vi "set ignition.vi"(10 "Ignition":bool, 11 "Array":T1[](array[typedef]) {"Data" format="%.0x"}) -> (3 "Array 2":T1[](array[typedef]) {"Data" format="%.0x"})   [LabVIEW 2021, in "uCanDriver.lvlib" / "uCAN.lvclass"]
uses:
  uCAN.lvclass
  typedefs/frame.ctl
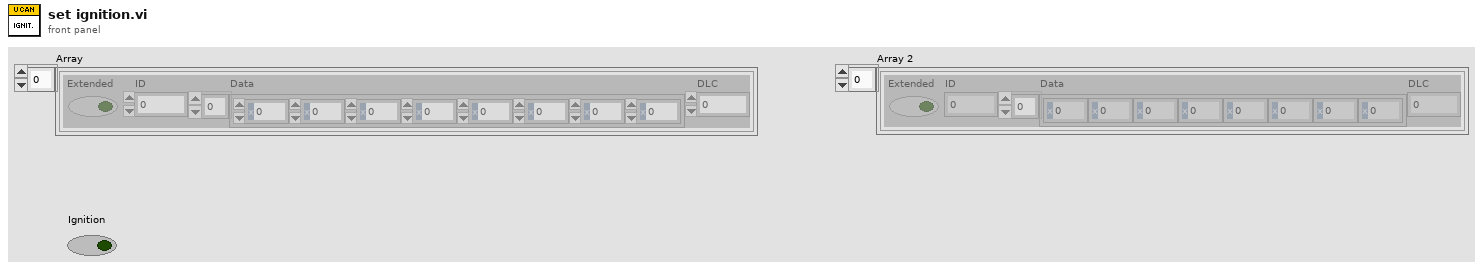
[diagram p1: front panel]
types:
  T1 = typedef "uCanDriver.lvlib/uCAN.lvclass/frame.ctl" = cluster{"Extended":bool, "ID":u32, "Data":u8[], "DLC":u8}
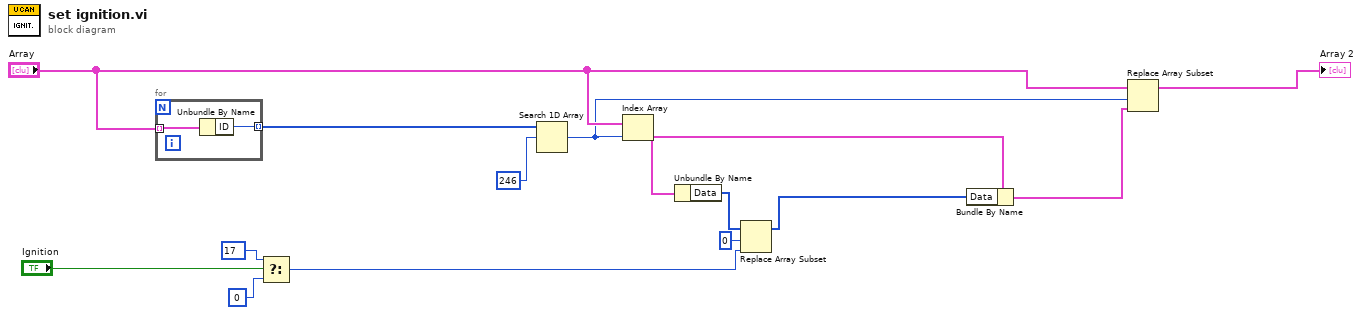
[diagram p0: block diagram]
diagram:
  n1 = for {
    tunnel: "Array" -> [w16] mode=indexing
    tunnel: [w15] -> w12 mode=indexing
    n2 = Unbundle By Name(w16) -> ("ID"=w15:u32)
  }
  n3 = Select(t=u32 17 ("element"), s="Ignition", f=u32 0 ("element")) -> (s? t:f=w2:u32)
  n4 = Search 1D Array(1D array=w12, element=u32 246) -> (index of element=w10:i32)  [unwired: 1 in]
  n5 = Index Array(array="Array", index=w10) -> (element=w14:T1)
  n6 = Unbundle By Name(w14) -> ("Data"=w7:u8[])
  n7 = Replace Array Subset(array=w7, new element=w2, index=0) -> (w6:u8[])
  n8 = Bundle By Name(cluster=w14, "Data"=w6) -> (w8:T1)
  n9 = Replace Array Subset(array="Array", new element=w8, index=w10) -> (→"Array 2":T1[])
